vi "clamps.vi"(10 "clamps":bool) -> ()   [LabVIEW 2014]
uses:
  <vilib>/Rock Robotics/WPI/Solenoid/WPI_SolenoidValue.ctl
  <vilib>/Rock Robotics/WPI/Solenoid/WPI_SolenoidGetEnum.vi
  <vilib>/Rock Robotics/WPI/Solenoid/WPI_SolenoidSetEnum.vi
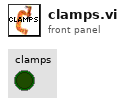
[diagram p1: front panel]
types:
  T1 = typedef "WPI_SolenoidValue.ctl" = enum16{"Off", "On", "Forward", "Reverse"}
  T2 = typedef "WPI_SolenoidDevRef.ctl" = cluster{"DevStatus":errorcluster, "Pneumatics Control Module":u8, "Forward Solenoid Channel":T3, "Reverse Solenoid Channel":T3}
  T3 = typedef "WPI_SolenoidChannel.ctl" = enum8{"Solenoid 0", "Solenoid 1", "Solenoid 2", "Solenoid 3", "Solenoid 4", "Solenoid 5", "Solenoid 6", "Solenoid 7", "Invalid"}
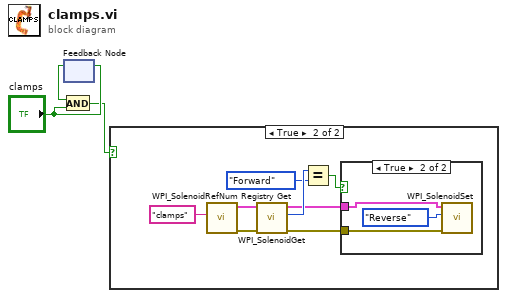
[diagram p0: block diagram]
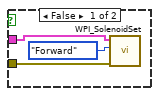
[diagram p3: hidden frame]
diagram:
  n1 = feedback-in #1("clamps") -> ()
  n2 = feedback #1() -> (w2:bool)  [unwired: 1 in]
  n3 = And(x=w2, y="clamps") -> (x .and. y?=w1:bool)
  n4 = case shown="True" w1 {
    frame False {
    }
    frame True {
      n5 = call <vilib>:"WPI_SolenoidRefNum Registry Get.vi"("refnum name"="clamps") -> ("error out"=w9:errorcluster, "SolenoidDevRef"=w10:T2)  [unwired: 9 in]
      n6 = call-poly <vilib>:"WPI_SolenoidGet.vi"("error in (no error)"=w9, "SolenoidDevRef"=w10) -> ("error out"=w4:errorcluster, "Value"=w8:T1, "SolenoidDevRef"=w5:T2)  [unwired: 7 in]
      n7 = Equal?(x=w8, y=WPI_SolenoidValue."Forward") -> (x = y?=w6:bool)
      n8 = case shown="True" w6 {
        tunnel: w5 -> [w13 w16]
        tunnel: w4 -> [w12 w15]
        frame False {
          n9 = call-poly <vilib>:"WPI_SolenoidSet.vi"("error in (no error)"=w12, "Value"=WPI_SolenoidValue."Forward", "SolenoidDevRef"=w13) -> ()  [unwired: 7 in, 2 out]
        }
        frame True {
          n10 = call-poly <vilib>:"WPI_SolenoidSet.vi"("error in (no error)"=w15, "Value"=WPI_SolenoidValue."Reverse", "SolenoidDevRef"=w16) -> ()  [unwired: 7 in, 2 out]
        }
      }
    }
  }
